vi "execute.vi"(8 "error in (no error)":errorcluster, 10 "Context in":refnum<class "Context.lvclass">, 11 "ShutdownCommand in":refnum<class "ShutdownCommand.lvclass">) -> (0 "error out":errorcluster, 2 "Context out":refnum<class "Context.lvclass">, 3 "ShutdownCommand out":refnum<class "ShutdownCommand.lvclass">)   [LabVIEW 2016, in "ShutdownCommand.lvclass"]
uses:
  ShutdownCommand.lvclass
  Context/Context.lvclass
  ShutdownCommand.lvclass/ShutdownCommand.ctl
  Context/Context.lvclass/Context.ctl
  Context/getModel.vi
  Context/setModel.vi
  Model/getState.vi
  States/State/State.lvclass
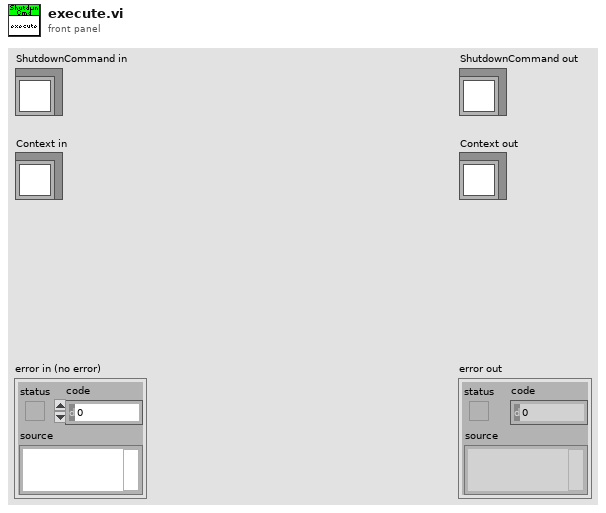
[diagram p1: front panel]
types:
  T1 = typedef "M1M3SupportTopics.lvlib/CommandShutdown.ctl" = cluster{"CommandId":T2, "Shutdown":bool}
  T2 = typedef "M1M3SupportTopics.lvlib/CommandId.ctl" = i32
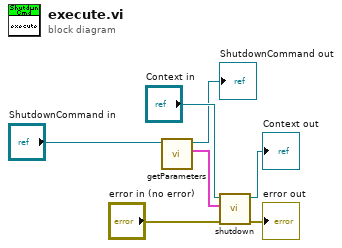
[diagram p0: block diagram]
diagram:
  n1 = call "getParameters.vi"("ShutdownCommand in"="ShutdownCommand in") -> ("Parameters"=w5:T1, "ShutdownCommand out"=→"ShutdownCommand out":refnum<class "ShutdownCommand.lvclass">)  [unwired: 9 in]
  n2 = call "shutdown.vi"("error in (no error)"="error in (no error)", "Parameters"=w5, "Context in"="Context in") -> ("error out"=→"error out":errorcluster, "Context out"=→"Context out":refnum<class "Context.lvclass">)  [unwired: 7 in]
